vi "Time.vi"(6 "Action (Get)":T1=enum."Get") -> (2 "Time [s]":sgl format="%.3g", 3 "Delta Time [s]":sgl format="%.3g")   [LabVIEW 2021]
uses:
  FGV Action.ctl
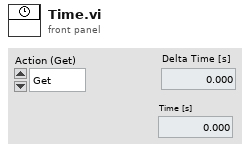
[diagram p1: front panel]
types:
  T1 = typedef "FGV Action.ctl" = enum16{"Set", "Get"}
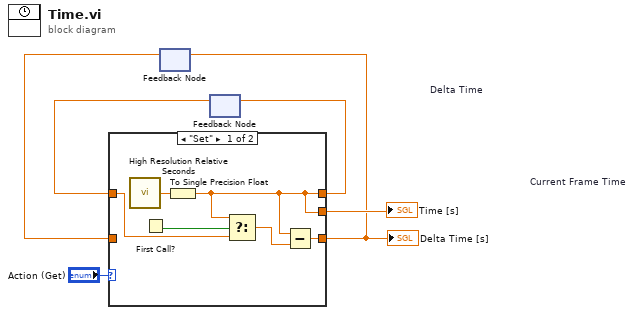
[diagram p0: block diagram]
diagram:
  n1 = feedback #1 "Delta Time"() -> (w3:sgl)  [unwired: 1 in]
  n2 = feedback #2 "Current Frame Time"() -> (w4:sgl)  [unwired: 1 in]
  n3 = case shown="\"Set\"" "Action (Get)" {
    tunnel: [w7 w14] -> w5
    tunnel: w4 -> [w8 w14]
    tunnel: [w12 w13] -> w1
    tunnel: w3 -> [_ w13]
    tunnel: [w7 w14] -> w2
    frame "Set" {
      n4 = call <vilib>:"High Resolution Relative Seconds.vi"() -> ("relative seconds"=w10:dbl)
      n5 = First Call?() -> (First Call?: T/F=w11:bool)
      n6 = To Single Precision Float(number=w10) -> (single precision float=w7:sgl)
      n7 = Select(t=w7, s=w11, f=w8) -> (s? t:f=w9:sgl)
      n8 = Subtract(x=w7, y=w9) -> (x-y=w12:sgl)
    }
    frame "Get" {
    }
  }
  "Time [s]" <- w2
  "Delta Time [s]" <- w1
  n9 = feedback-in #1(w1) -> ()
  n10 = feedback-in #2(w5) -> ()
